vi "FGGA Serial Data Server & Recordingv4.0.vi"() -> ()   [LabVIEW 2014]
uses:
  <vilib>/Instr/_visa.llb/VISA Set IO Buffer Mask.ctl
  <vilib>/Instr/_visa.llb/VISA Flush IO Buffer Mask.ctl
  <vilib>/Platform/TimedLoop/XDataNode/timing_clust.ctl
  <vilib>/Platform/TimedLoop/XDataNode/nitl_modes.ctl
  <vilib>/Platform/TimedLoop/XDataNode/wakeup.ctl
  C:/Program Files (x86)/National Instruments/LabVIEW 2014/examples/Data Communication/Network Streams/Simple Network Streams/support/Network Stream Command.ctl
  <vilib>/Utility/error.llb/whitespace.ctl
  <vilib>/Instr/_visa.llb/VISA Configure Serial Port (Instr).vi
  <vilib>/Utility/tcp.llb/UDP Multicast Write-Only Open.vi
  <vilib>/platform/TimedLoop/XDataNode/XDataNode.xnode
  <vilib>/Platform/TimedLoop/XDataNode/XDNodeRunTimeDep.lvlib
panel:
  out "FGGA Pump":bool
  out "Flight Number":string
  out "Stop File Write":bool
  out "Default file name":string
  out "MFC":dbl[](array[numeric])
  out "FGGA restart":bool
  out "V4":bool
  out "V3":bool
  out "V2":bool
  out "V1":bool
  out "error out 2":errorcluster
  out "error out":errorcluster
  in  "MFC_1 SLPM set value":dbl
  out "Value Read":string
  out "status":bool
  in  "VISA resource name":refnum<visa-resource-name>="ASRL3::INSTR"
  in  "timeout (10sec) 2":u32=3000
  out "Labview_Viewer_UDP_Error_Out":errorcluster
  in  "Clear Display\nErrors":bool
  out "Data Processing":bool
  out "TCP Binary Packet":string
  out "UDP Time Stamp Offset":i32=1
  out "Data String":string
  out "UDP_ACSII_Out":string
  out "Serial error out":errorcluster
  out "SEPTIC TCP Error Out":errorcluster
  out "TCP packet\nSend To SEPTIC":bool
  out "FISH TCP Error Out":errorcluster
  out "TCP packet\nSend To FISH":bool
  out "UDP_Pack_num":u32
  out "UDP_Out Status":bool
  out "UDP_Out_Error Out":errorcluster
  out "Data Array":string[](array[string])
  out "RAW DATA":string
  in  "stop":bool
  in  "timeout (10sec)":u32=1500
  in  "VISA resource name":refnum<visa-resource-name>="ASRL7::INSTR"
  out "Number of times \nRead time out":u32
  out "Loop count":i32
  # "Date"
  # "Time"
  # "CH4"
  # "CO2"
  # "H2O"
  # "Cell Pressure"
  # "Cell Temperature"
  # "Spectral Flag"
  # "Ring Down Time (Laser A)"
  # "Ring Down Time (Laser B)"
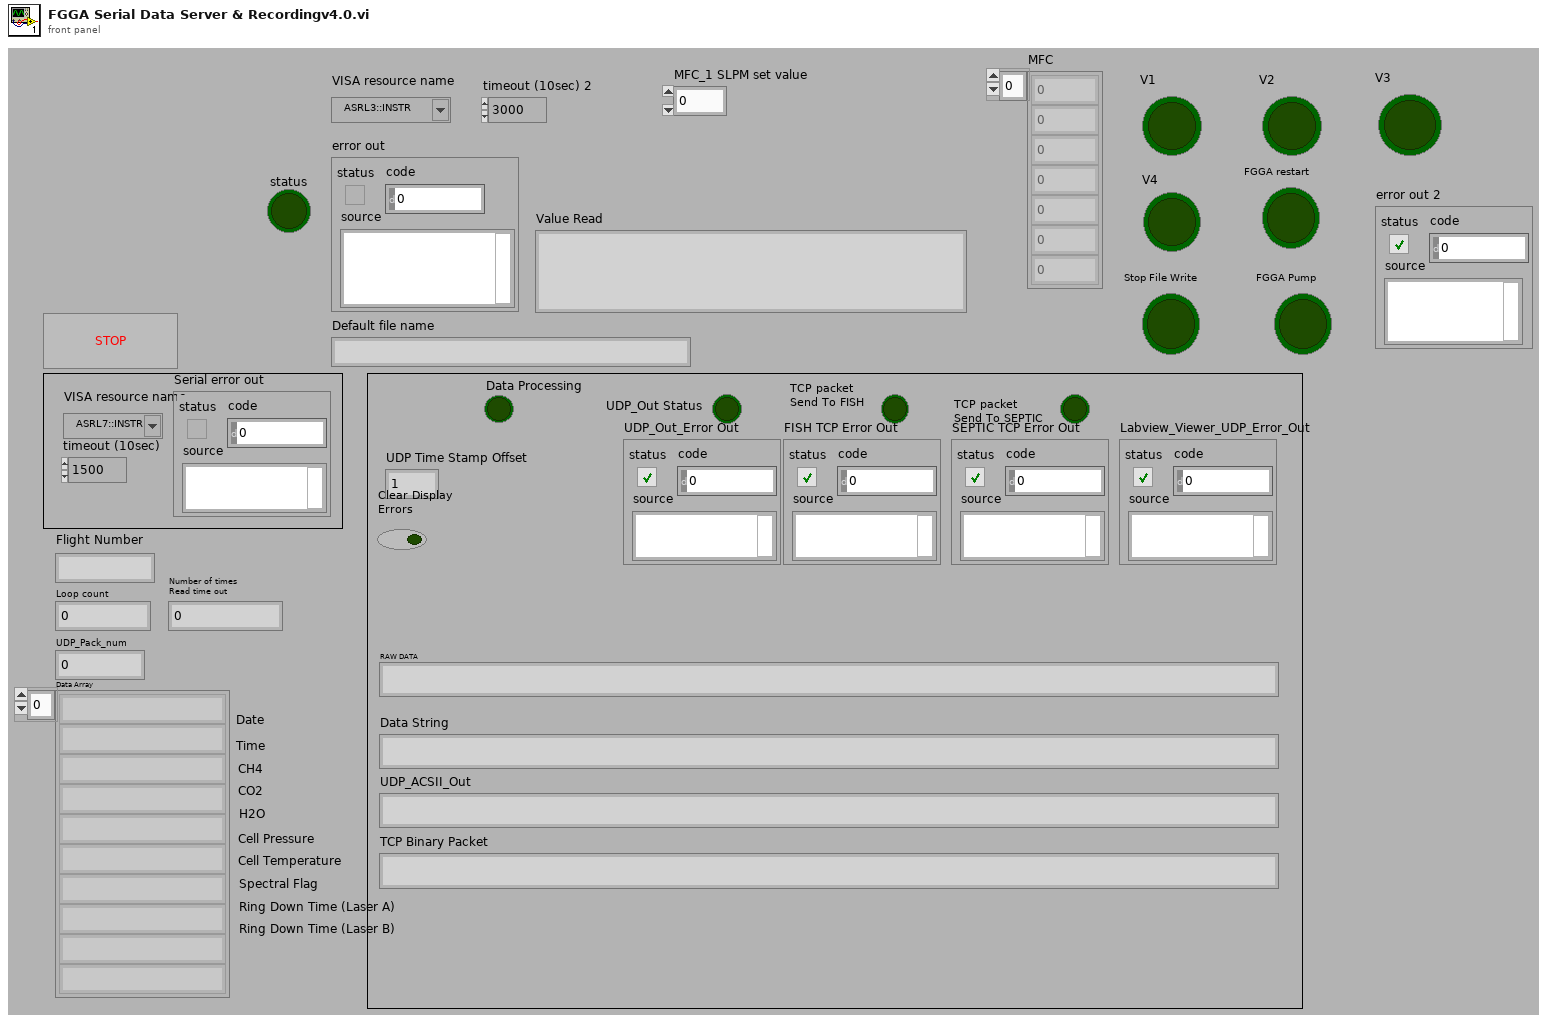
[diagram p1: front panel]
types:
  T1 = typedef "VISA Flush IO Buffer Mask.ctl" = u16
  T2 = typedef "VISA Set IO Buffer Mask.ctl" = u16
  T3 = typedef "XDNodeRunTimeDep.lvlib/timing_clust.ctl" = cluster{"Expected End [f-1]":u64, "Actual End [f-1]":u64, "Finished Late? [f-1]":bool, "Expected End [i-1]":u64, "Actual End [i-1]":u64, "Finished Late? [i-1]":bool, "Expected Start [i]":u64, "Actual Start [i]":u64, "Expected Start [f]":u64, "Actual Start [f]":u64, "Source Name":string, "Structure Name":string, "Period":i64, "Deadline":i64, "Offset":i64, "Start":i64, "Priority":i32, "Timeout":i32, "Mode":T4, "Wakeup Reason":T5, "Error":errorcluster, "Source Type":string, "Secondary Source Type":string, "Global End Time":u64, "Global Start Time":u64, "Frame Duration":u64, "Iteration Duration":u64, "Assigned CPU":i32, "I/O Scan Engine Mode":u32}
  T4 = typedef "XDNodeRunTimeDep.lvlib/nitl_modes.ctl" = enum32{"No Change", "Process missed periods, maintain original phase", "Discard missed periods, maintain original phase", "Process missed periods, ignore original phase", "Discard missed periods, ignore original phase"}
  T5 = typedef "XDNodeRunTimeDep.lvlib/wakeup.ctl" = enum32{"Normal", "Aborted", "Asynchronous wakeup", "Timing source error", "Timed loop error", "Timeout"}
  T6 = typedef "Network Stream Command.ctl" = cluster{"Message":string, "Message Data":variant}
  T7 = enum16{"open", "replace", "create", "open or create", "replace or create", "replace or create with confirmation"}
  T8 = typedef "whitespace.ctl" = u16
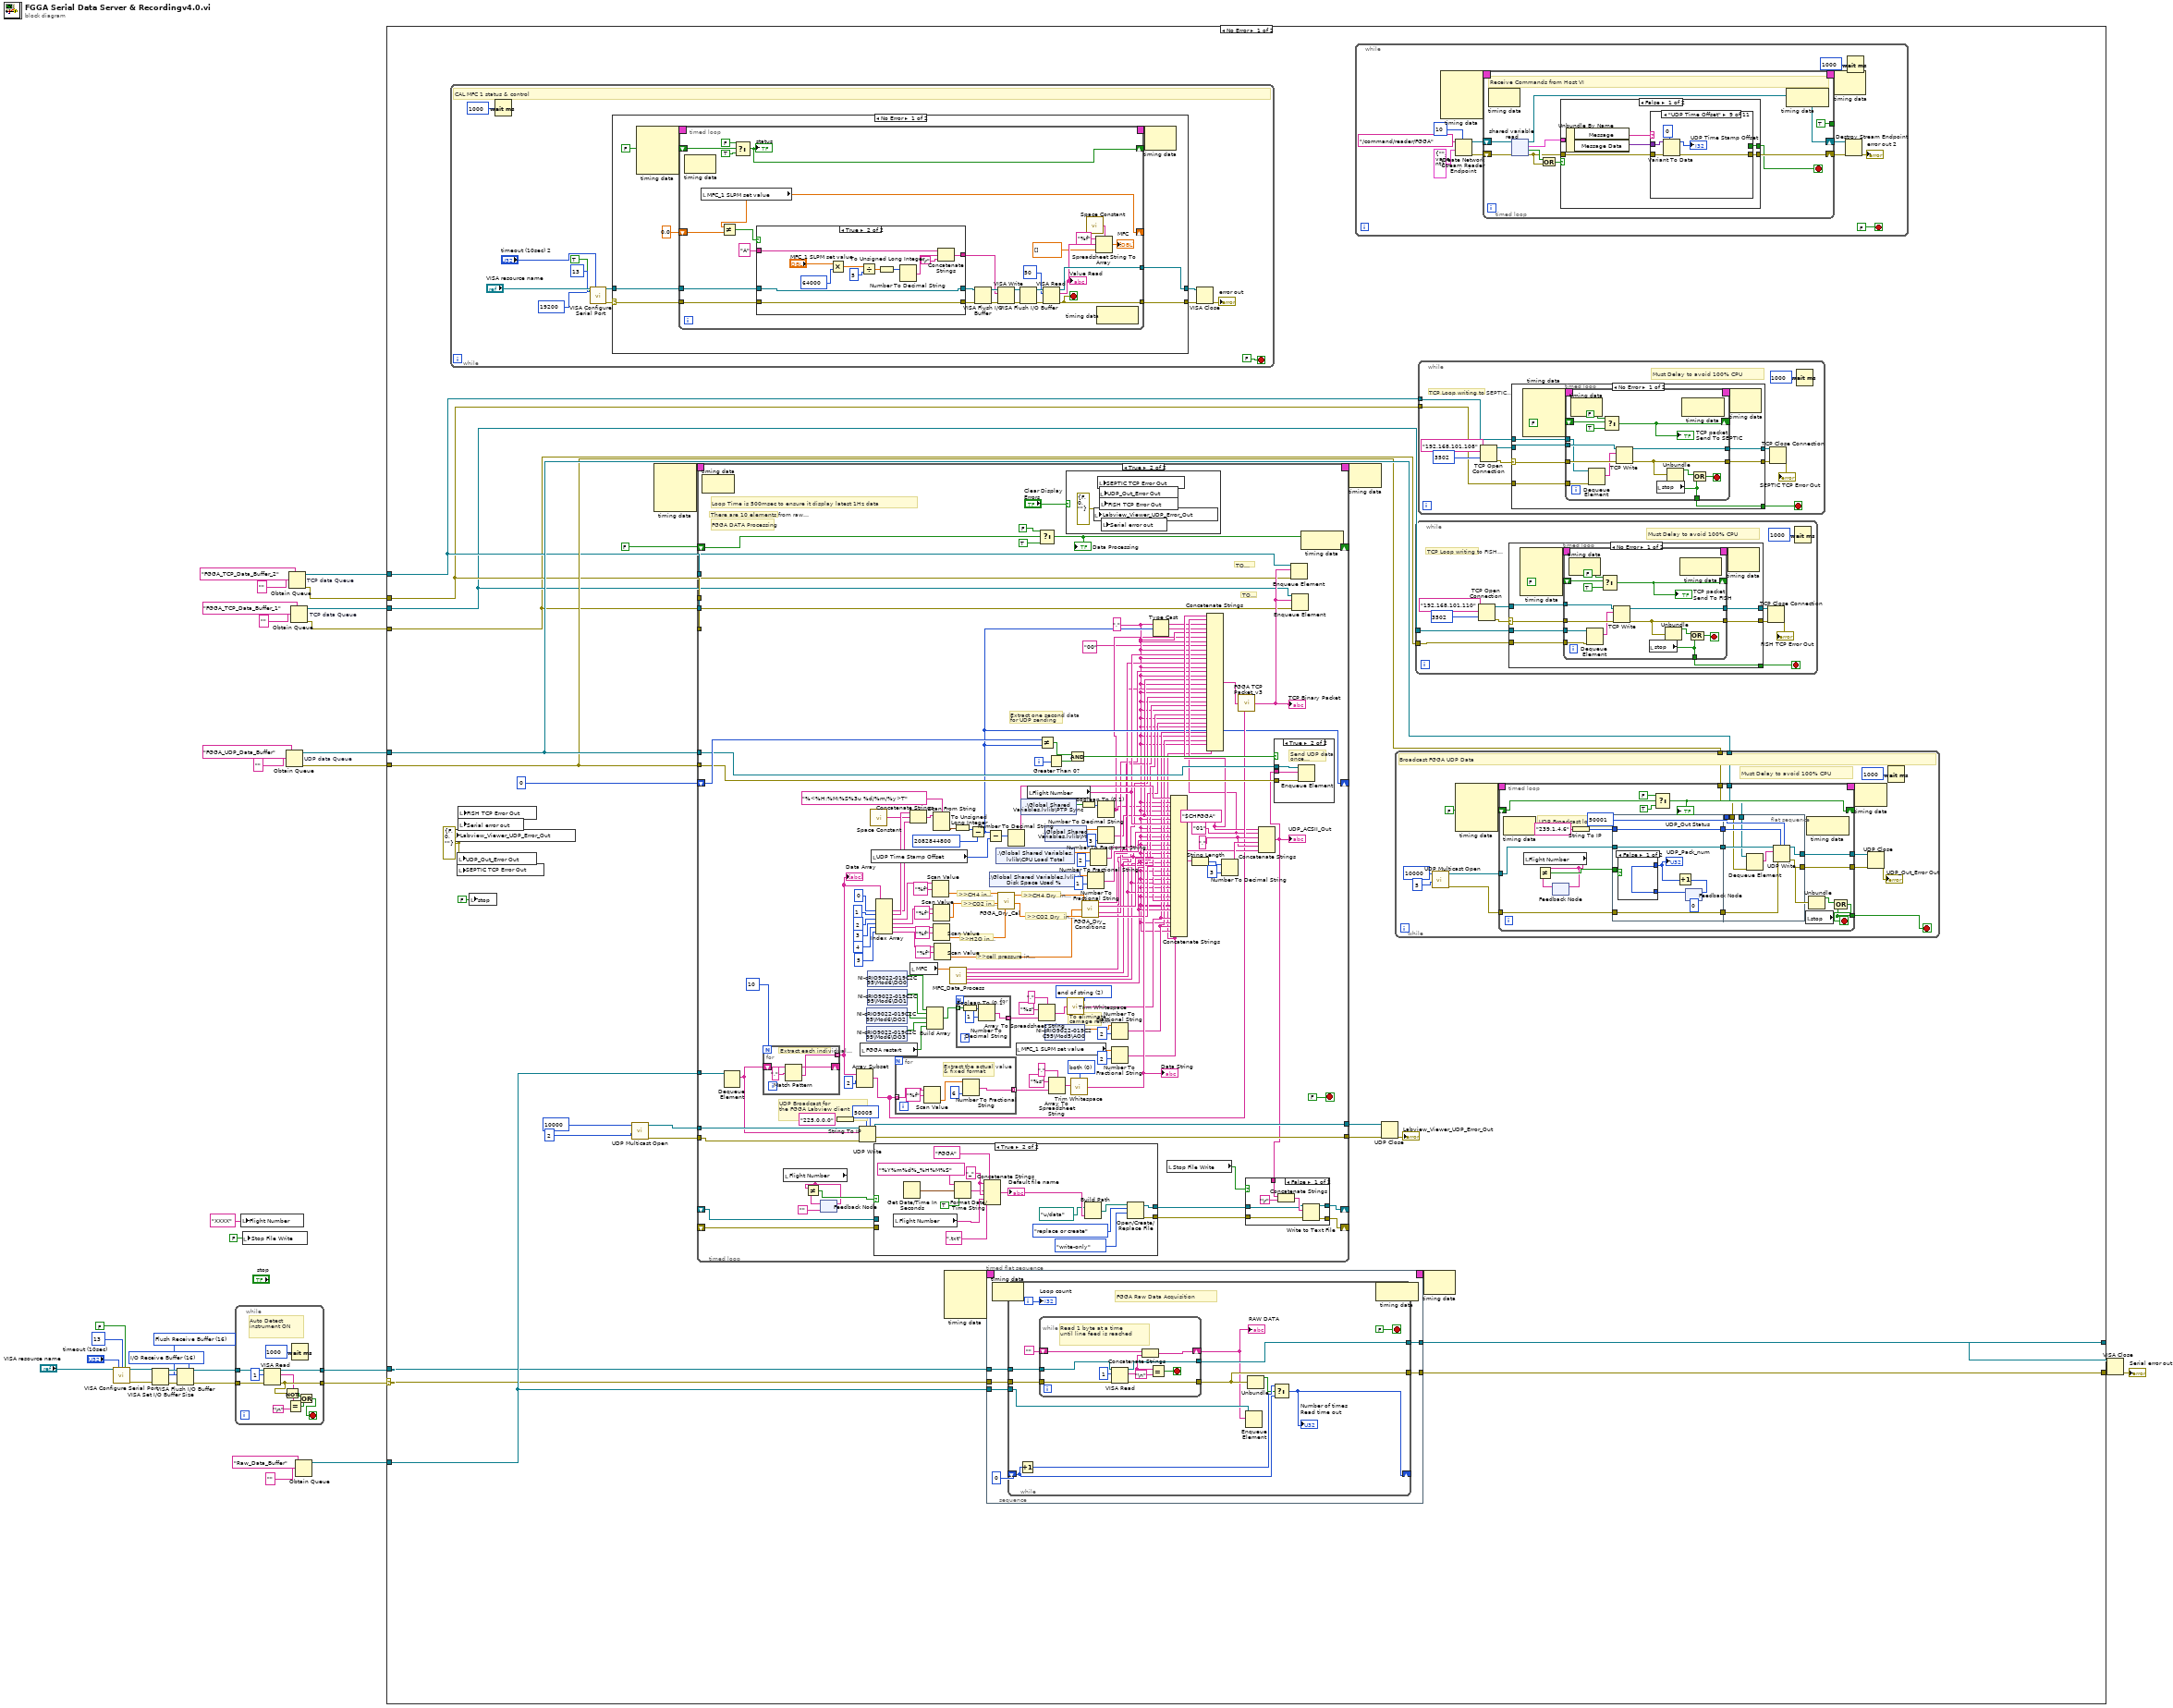
[diagram p0: block diagram]
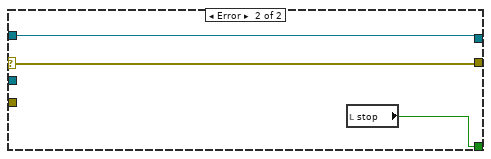
[diagram p2: hidden frame]
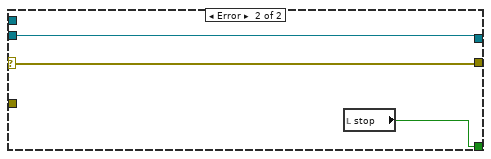
[diagram p3: hidden frame]
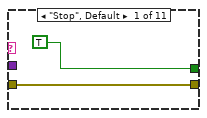
[diagram p4: hidden frame]
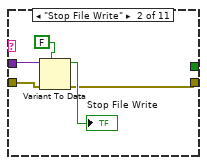
[diagram p5: hidden frame]
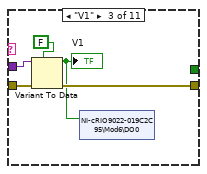
[diagram p6: hidden frame]
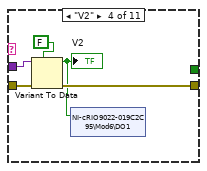
[diagram p7: hidden frame]
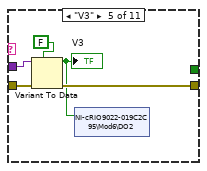
[diagram p8: hidden frame]
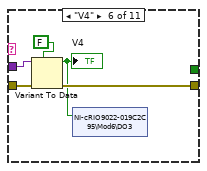
[diagram p9: hidden frame]
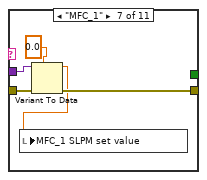
[diagram p10: hidden frame]
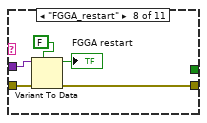
[diagram p11: hidden frame]
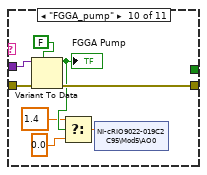
[diagram p12: hidden frame]
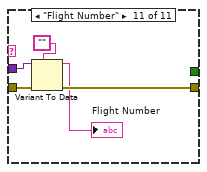
[diagram p13: hidden frame]
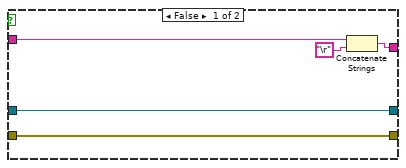
[diagram p15: hidden frame]
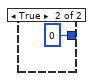
[diagram p17: hidden frame]
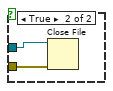
[diagram p19: hidden frame]
diagram:
  w9 = T1 16 items=["Flush Receive Buffer"=16, "Write Transmit Buffer to Device"=32, "Flush Receive Buffer (No I/O)"=64, "Flush Transmit Buffer"=128] ("Mask")
  w10 = T2 16 items=["I/O Receive Buffer"=16, "I/O Transmit Buffer"=32, "I/O Receive and Transmit Buffer"=48] ("Mask")
  n1 = call-poly "VISA Configure Serial Port"("VISA resource name"="VISA resource name", "timeout (10sec)"="timeout (10sec)", "termination char\n(0xA = '\\n' = LF)"=u8 13 ("termination char\n(0xA = '\\n' = LF)"), "Enable Termination\nChar (T)"=FALSE ("Enable Termination\nChar (T)")) -> ("VISA resource name out"=w8:refnum<visa-resource-name>, "error out"=w7:errorcluster)  [unwired: 10 in]
  n2 = VISA Set I/O Buffer Size(VISA resource name=w8, mask (16)=w10, error in (no error)=w7) -> (VISA resource name out=w11:refnum<visa-resource-name>, error out=w12:errorcluster)  [unwired: 1 in]
  n3 = VISA Flush I/O Buffer(VISA resource name=w11, mask (16)=w9, error in (no error)=w12) -> (VISA resource name out=w6:refnum<visa-resource-name>, error out=w5:errorcluster)
  n4 = while {
    tunnel: w6 -> [w45]
    tunnel: w5 -> [w44]
    tunnel: [w42] -> w4
    tunnel: [w41] -> w3
    stop <- w36 stop-if-true
    # "Auto Detect\ninstrument ON"
    n5 = VISA Read(VISA resource name=w45, byte count=u32 1, error in (no error)=w44) -> (VISA resource name out=w41:refnum<visa-resource-name>, read buffer=w39:string, error out=w42:errorcluster)  [unwired: 1 out]
    n6 = Not(x=w42) -> (.not. x?=w38:bool)
    n7 = Equal?(x=w39, y="\n") -> (x = y?=w37:bool)
    n8 = Wait (ms)(milliseconds to wait=u32 1000) -> ()  [unwired: 1 out]
    n9 = Or(x=w38, y=w37) -> (x .or. y?=w36:bool)
  }
  n10 = local write "Flight Number"("XXXX" ("Flight Number")) -> ()
  n11 = local write "Stop File Write"(FALSE ("Stop File Write")) -> ()
  n12 = Obtain Queue "UDP data Queue"(name (unnamed)="FGGA_UDP_Data_Buffer", element data type="") -> (queue out=w22:refnum<queue>, error out=w21:errorcluster)  [unwired: 3 in, 1 out]
  n13 = Obtain Queue "TCP data Queue"(name (unnamed)="FGGA_TCP_Data_Buffer_2", element data type="") -> (queue out=w16:refnum<queue>, error out=w15:errorcluster)  [unwired: 3 in, 1 out]
  n14 = Obtain Queue "TCP data Queue"(name (unnamed)="FGGA_TCP_Data_Buffer_1", element data type="") -> (queue out=w14:refnum<queue>, error out=w13:errorcluster)  [unwired: 3 in, 1 out]
  n15 = Obtain Queue(name (unnamed)="Raw_Data_Buffer", element data type="") -> (queue out=w28:refnum<queue>)  [unwired: 3 in, 2 out]
  n16 = case shown="No Error" w4 {
    selector: w4 -> [w48 w592]
    tunnel: w3 -> [w49 w593]
    tunnel: [w70 w593] -> w25
    tunnel: [w71 w592] -> w26
    tunnel: w28 -> [w67 _]
    tunnel: w22 -> [w65 _]
    tunnel: w21 -> [w64 _]
    tunnel: w16 -> [w63 _]
    tunnel: w15 -> [w62 _]
    tunnel: w14 -> [w61 _]
    tunnel: w13 -> [w60 _]
    frame No Error {
      w51 = errorcluster {"status"=FALSE, "code"=0, "source"=""} ("UDP Error Out")
      n17 = while {
        stop <- FALSE stop-if-true
        # "CAL MFC 1 status & control"
        n18 = Wait (ms)(milliseconds to wait=u32 1000) -> ()  [unwired: 1 out]
        n19 = call-poly "VISA Configure Serial Port"("VISA resource name"="VISA resource name", "timeout (10sec)"="timeout (10sec) 2", "termination char\n(0xA = '\\n' = LF)"=u8 13 ("termination char\n(0xA = '\\n' = LF)"), "Enable Termination\nChar (T)"=TRUE ("Enable Termination\nChar (T)"), "baud rate (9600)"=u32 19200) -> ("VISA resource name out"=w294:refnum<visa-resource-name>, "error out"=w290:errorcluster)  [unwired: 9 in]
        n20 = case shown="No Error" w290 {
          selector: w290 -> [w301 w351]
          tunnel: w294 -> [w302 w352]
          tunnel: [w300 w352] -> w293
          tunnel: [w299 w351] -> w292
          frame No Error {
            n21 = node-c288() -> (w297:T3)  [unwired: 4 in]
            n22 = timed-loop {
              tunnel: w302 -> [w325]
              tunnel: w301 -> [w323]
              tunnel: [w316] -> w300
              tunnel: [w311] -> w299
              shift-right: [w312] -> _
              shift-left: FALSE -> [w315]
              timing: w297 -> [_]
              timing-out: [_] -> w296
              shift-right: [w303] -> _
              shift-left: 0.0 -> [w305]
              stop <- w311 stop-if-true
              n23 = node-c288() -> ()  [unwired: 1 in, 1 out]
              n24 = local read "MFC_1 SLPM set value"() -> (w303:dbl)
              n25 = Not Equal?(x=w303, y=w305) -> (x != y?=w304:bool)
              n26 = Select(t=FALSE, s=w315, f=TRUE) -> (s? t:f=w312:bool)
              "status" <- w312
              n27 = case shown="True" w304 {
                tunnel: w325 -> [w333 w348]
                tunnel: [w333 w348] -> w324
                tunnel: w323 -> [w332 w347]
                tunnel: [w332 w347] -> w322
                tunnel: "A" -> [w336 w340]
                tunnel: [w334 w337] -> w320
                frame False {
                  n28 = Concatenate Strings(w336, "\r") -> (w334:string)
                }
                frame True {
                  n29 = Multiply(x="MFC_1 SLPM set value", y=u32 64000) -> (x*y=w344:dbl)
                  n30 = Divide(x=w344, y=u32 5) -> (x/y=w342:dbl)
                  n31 = To Unsigned Long Integer(number=w342) -> (unsigned 32bit integer=w341:u32)
                  n32 = Number To Decimal String(number=w341) -> (decimal integer string=w339:string)  [unwired: 1 in]
                  n33 = Concatenate Strings(w340, w339, "\r") -> (w337:string)
                }
              }
              n34 = VISA Flush I/O Buffer(VISA resource name=w324, error in (no error)=w322) -> (VISA resource name out=w327:refnum<visa-resource-name>, error out=w326:errorcluster)  [unwired: 1 in]
              n35 = VISA Write(VISA resource name=w327, write buffer=w320, error in (no error)=w326) -> (VISA resource name out=w319:refnum<visa-resource-name>, error out=w318:errorcluster)  [unwired: 1 out]
              n36 = VISA Flush I/O Buffer(VISA resource name=w319, error in (no error)=w318) -> (VISA resource name out=w329:refnum<visa-resource-name>, error out=w328:errorcluster)  [unwired: 1 in]
              n37 = VISA Read(VISA resource name=w329, byte count=u32 50, error in (no error)=w328) -> (VISA resource name out=w316:refnum<visa-resource-name>, read buffer=w310:string, error out=w311:errorcluster)  [unwired: 1 out]
              "Value Read" <- w310
              n38 = call <vilib>:"Space Constant.vi"() -> ("String"=w309:string)
              n39 = Spreadsheet String To Array(delimiter (Tab)=w309, format string="%f", spreadsheet string=w310, array type (2D Dbl)=dbl[] []) -> (array=→"MFC":dbl[])
              n40 = node-c288() -> ()  [unwired: 1 in, 1 out]
            }
            n41 = node-c288(w296) -> ()  [unwired: 1 out]
          }
          frame Error {
          }
        }
        n42 = VISA Close(VISA resource name=w293, error in (no error)=w292) -> (error out=→"error out":errorcluster)
      }
      n43 = local write "Labview_Viewer_UDP_Error_Out"(w51) -> ()
      n44 = local write "UDP_Out_Error Out"(w51) -> ()
      n45 = local write "SEPTIC TCP Error Out"(w51) -> ()
      n46 = local write "FISH TCP Error Out"(w51) -> ()
      n47 = local write "Serial error out"(w51) -> ()
      n48 = local write "stop"(FALSE ("stop")) -> ()
      n49 = call-poly <vilib>:"UDP Multicast Open.vi"("time-to-live (1)"=u16 2, "port"=u16 10000) -> ("error out"=w55:errorcluster, "connection ID"=w56:refnum<k16>)  [unwired: 8 in]
      n50 = node-c288() -> (w69:T3)  [unwired: 4 in]
      n51 = timed-loop {
        timing: w69 -> [_]
        timing-out: [_] -> w68
        tunnel: w67 -> [w544]
        tunnel: w65 -> [w500]
        tunnel: w64 -> [w499]
        shift-right: [w429] -> _
        shift-left: u32 0 -> [w503]
        tunnel: w63 -> [w496]
        tunnel: w62 -> [w495]
        tunnel: w61 -> [w494]
        tunnel: w60 -> [w493]
        shift-right: [w489] -> _
        shift-left: FALSE -> [w492]
        tunnel: w56 -> [w485]
        tunnel: w55 -> [w484]
        tunnel: [w483] -> w54
        tunnel: [w482] -> w53
        shift-right: [w469] -> _
        shift-left: _ -> [w461]
        shift-right: [w459] -> _
        shift-left: _ -> [w460]
        i -> [w502]
        stop <- FALSE stop-if-true
        w433 = T8 2 items=["both", "start of string", "end of string"] ("location (both)")
        w416 = ","
        w530 = T8 0 items=["both", "start of string", "end of string"] ("location (both)")
        w538 = ","
        w430 = "01"
        w431 = "$CHFGGA"
        # "To eliminate\ncarriage return"
        # ">>cell pressure in torr>>"
        # "UDP Broadcast for\nthe FGGA Labview client"
        # "There are 10 elements from raw packet"
        # "TO SEPTIC"
        # "TO FISH"
        # "Extract one second data\nfor UDP sending"
        # ">>CO2 Dry  in ppm>>"
        # ">>CH4 Dry  in ppb>>"
        # ">>H2O in ppm>>"
        # ">>CO2 in ppm>>"
        # ">>CH4 in ppm>>"
        # "Loop Time is 500msec to ensure it display latest 1Hz data"
        # "FGGA DATA Processing"
        n52 = node-c288() -> ()  [unwired: 1 in, 1 out]
        n53 = Dequeue Element(queue=w544) -> (element=w481:string)  [unwired: 2 in, 3 out]
        n54 = for {
          N: 10 -> [_]
          shift-right: [w586] -> _
          shift-left: w481 -> [w584]
          tunnel: [w585] -> w535 mode=indexing
          # "Extract each individual param"
          n55 = Match Pattern(string=w584, regular expression=",") -> (before substring=w585:string, after substring=w586:string)  [unwired: 1 in, 2 out]
        }
        "Data Array" <- w535
        n56 = local read "Flight Number"() -> (w458:string)
        n57 = feedback #1("" ("Flight Number")) -> (w466:string)
        n58 = Not Equal?(x=w458, y=w466) -> (x != y?=w464:bool)
        n59 = feedback-in #1(w458) -> ()
        n60 = String To IP(1:"225.0.0.0" ("name")) -> (0:w486:u32)
        n61 = Array Subset(array=w535, index=2) -> (w498:string[])  [unwired: 1 in]
        n62 = UDP Write(address=w486, port or service name=u16 50005, connection ID=w485, data in=w481, 8:w484) -> (error out=w482:errorcluster, 3:w483:refnum<k16>)  [unwired: 1 in]
        n63 = local read "FGGA restart"() -> (w443:bool)
        n64 = shared-variable "NI-cRIO9022-019C2C95\\Mod6\\DO2"() -> (w449:bool)  [unwired: 1 in, 1 out]
        n65 = shared-variable "NI-cRIO9022-019C2C95\\Mod6\\DO3"() -> (w448:bool)  [unwired: 1 in, 1 out]
        n66 = shared-variable "NI-cRIO9022-019C2C95\\Mod6\\DO0"() -> (w451:bool)  [unwired: 1 in, 1 out]
        n67 = shared-variable "NI-cRIO9022-019C2C95\\Mod6\\DO1"() -> (w450:bool)  [unwired: 1 in, 1 out]
        n68 = call <vilib>:"Space Constant.vi"() -> ("String"=w513:string)
        n69 = local read "UDP Time Stamp Offset"() -> (w432:i32)
        n70 = case shown="True" w464 {
          tunnel: [w550 w552] -> w463
          tunnel: [w549 w551] -> w462
          tunnel: w461 -> [w550 _]
          tunnel: w460 -> [w549 _]
          frame False {
          }
          frame True {
            w558 = "_" ("string")
            n71 = local read "Flight Number"() -> (w565:string)
            n72 = Get Date/Time In Seconds() -> (seconds since 1Jan1904=w553:timestamp)
            n73 = Format Date/Time String(time format string (%c)="%Y%m%d%_%H%M%S", seconds (now)=w553, UTC format=TRUE) -> (date/time string=w555:string)
            n74 = Concatenate Strings("FGGA" ("string"), w558, w555, w558, w565, ".txt" ("string")) -> (w560:string)
            "Default file name" <- w560
            n75 = Build Path(base path=path "u:/data", name or relative path=w560) -> (appended path=w564:path)
            n76 = Open/Create/Replace File(file path (use dialog)=w564, operation (0:open)=T7."replace or create", access (0:read/write)=enum16{"read/write", "read-only", "write-only"}."write-only") -> (refnum out=w552:refnum<file>, error out=w551:errorcluster)  [unwired: 3 in, 1 out]
          }
        }
        n77 = Index Array(array=w535, index #1=0 ("index"), index #2=1 ("index"), index #3=2 ("index"), index #4=3 ("index"), index #5=4 ("index"), index #6=5 ("index")) -> (element #1=w512:string, element #2=w514:string, element #3=w518:string, element #4=w517:string, element #5=w516:string, element #6=w474:string)
        n78 = for {
          tunnel: w498 -> [w582] mode=indexing
          tunnel: [w579] -> w528 mode=indexing
          # "Extract the actual value\n& fixed format"
          n79 = Scan Value(string=w582, format string="%f") -> (value=w580:dbl)  [unwired: 1 in, 1 out]
          n80 = Number To Fractional String(number=w580, precision (6)=i16 6) -> (F-format string=w579:string)  [unwired: 2 in]
        }
        n81 = Concatenate Strings(w514, w513, w512) -> (w511:string)
        n82 = local read "MFC"() -> (w470:dbl[])
        n83 = Build Array(w451, w450, w449, w448, w443) -> (w447:bool[])
        n84 = Scan Value(string=w518, format string="%f") -> (value=w520:dbl)  [unwired: 1 in, 1 out]
        n85 = Scan Value(string=w517, format string="%f") -> (value=w519:dbl)  [unwired: 1 in, 1 out]
        n86 = Scan From String(format string="%<%H:%M:%S%3u %d/%m/%y>T", input string=w511) -> (output 1=w508:timestamp)  [unwired: 3 in, 3 out]
        n87 = Scan Value(string=w516, format string="%f") -> (value=w471:dbl)  [unwired: 1 in, 1 out]
        n88 = Scan Value(string=w474, format string="%f") -> (value=w472:dbl)  [unwired: 1 in, 1 out]
        n89 = call "MFC_Data_Process.vi"("MFC"=w470) -> ("MFC Absolute Pressure"=w423:string, "MFC Temperature"=w422:string, "MFC Volumetric Flow"=w421:string, "MFC Mass Flow"=w420:string, "MFC Set Point"=w419:string)  [unwired: 10 in]
        n90 = To Unsigned Long Integer(number=w508) -> (unsigned 32bit integer=w509:u32)
        n91 = for {
          tunnel: w447 -> [w547] mode=indexing
          tunnel: [w546] -> w444 mode=indexing
          n92 = Boolean To (0,1)(Boolean=w547) -> (0, 1=w548:i16)
          n93 = Number To Decimal String(number=w548, width (-)=i16 1) -> (decimal integer string=w546:string)
        }
        n94 = Subtract(x=w509, y=u32 2082844800) -> (x-y=w429:u32)
        n95 = Subtract(x=w429, y=w432) -> (x-y=w506:u32)
        n96 = shared-variable ".\\Global Shared Variables.lvlib\\Disk Space Used %"() -> (w436:dbl)  [unwired: 1 in, 1 out]
        n97 = shared-variable ".\\Global Shared Variables.lvlib\\CPU Load Total"() -> (w457:dbl)  [unwired: 1 in, 1 out]
        n98 = call "FGGA_Dry_Cal.vi"("H2O"=w471, "CO2_Wet"=w519, "CH4_Wet"=w520) -> ("CO2_Dry"=w476:dbl, "CH4_Dry"=w478:dbl)  [unwired: 7 in]
        n99 = Number To Decimal String(number=w506) -> (decimal integer string=w507:string)  [unwired: 1 in]
        n100 = local read "MFC_1 SLPM set value"() -> (w439:dbl)
        n101 = shared-variable ".\\Global Shared Variables.lvlib\\PTP Sync"() -> (w452:bool)  [unwired: 1 in, 1 out]
        n102 = local read "Flight Number"() -> (w427:string)
        n103 = Array To Spreadsheet String(delimiter (Tab)=",", array=w444, 3:"%s" ("format string")) -> (spreadsheet string=w434:string)
        n104 = Select(t=FALSE, s=w492, f=TRUE) -> (s? t:f=w489:bool)
        "Data Processing" <- w489
        n105 = Not Equal?(x=w503, y=w429) -> (x != y?=w504:bool)
        n106 = shared-variable ".\\Global Shared Variables.lvlib\\MFM"() -> (w455:dbl)  [unwired: 1 in, 1 out]
        n107 = shared-variable "NI-cRIO9022-019C2C95\\Mod5\\AO0"() -> (w441:dbl)  [unwired: 1 in, 1 out]
        n108 = Greater Than 0?(x=w502) -> (x > 0?=w505:bool)
        n109 = Array To Spreadsheet String(delimiter (Tab)=",", array=w528, 3:"%s" ("format string")) -> (spreadsheet string=w529:string)
        n110 = case shown="True" "Clear Display\nErrors" {
          frame False {
          }
          frame True {
            w575 = errorcluster {"status"=FALSE, "code"=0, "source"=""} ("UDP Error Out")
            n111 = local write "Labview_Viewer_UDP_Error_Out"(w575) -> ()
            n112 = local write "SEPTIC TCP Error Out"(w575) -> ()
            n113 = local write "UDP_Out_Error Out"(w575) -> ()
            n114 = local write "FISH TCP Error Out"(w575) -> ()
            n115 = local write "Serial error out"(w575) -> ()
          }
        }
        n116 = call <vilib>:"Trim Whitespace.vi"("string"=w434, "location (both)"=w433) -> ("trimmed string"=w418:string)
        n117 = call <vilib>:"Trim Whitespace.vi"("string"=w529, "location (both)"=w530) -> ("trimmed string"=w527:string)
        "Data String" <- w527
        n118 = Compound Arithmetic op=AND(w504, w505) -> (w501:bool)
        n119 = Boolean To (0,1)(Boolean=w452) -> (0, 1=w453:i16)
        n120 = call "FGGA_Dry_Conditions.vi"("CH4_Dry"=w478, "Pressure"=w472, "CO2_Dry"=w476) -> ("CH4_Dry_TCP"=w426:string, "CH4_Dry_UDP"=w480:string, "CO2_Dry_TCP"=w425:string, "CO2_Dry_UDP"=w479:string)  [unwired: 9 in]
        n121 = Number To Fractional String(number=w436, precision (6)=i16 1) -> (F-format string=w435:string)  [unwired: 2 in]
        n122 = Number To Fractional String(number=w457, precision (6)=i16 2) -> (F-format string=w438:string)  [unwired: 2 in]
        n123 = Number To Decimal String(number=w453) -> (decimal integer string=w413:string)  [unwired: 1 in]
        n124 = Number To Fractional String(number=w455, precision (6)=i16 3) -> (F-format string=w424:string)  [unwired: 2 in]
        n125 = Number To Fractional String(number=w441, precision (6)=i16 2) -> (F-format string=w417:string)  [unwired: 2 in]
        n126 = Number To Fractional String(number=w439, precision (6)=i16 2) -> (F-format string=w415:string)  [unwired: 2 in]
        n127 = Type Cast(x=w429) -> (*(type *) &x=w428:string)  [unwired: 1 in]
        n128 = local read "Stop File Write"() -> (w467:bool)
        n129 = Concatenate Strings(w507, w416, w413, w416, w424, w416, w427, w416, w438, w416, w435, w416, w527, w416, w480, w416, w479, w416, w423, w416, w422, w416, w421, w416, w420, w416, w419, w416, w418, w416, w417, w416, w415) -> (w537:string)
        n130 = String Length(string=w537) -> (length=w541:i32)
        n131 = Concatenate Strings(w431, w430, w416, w428, w416, w413, w416, "00", w416, w427, w416, w426, w416, w425, w416, w424, w416, w423, w416, w422, w416, w421, w416, w420, w416, w419, w416, w418, w416, w417, w416, w415) -> (w414:string)
        n132 = Number To Decimal String(number=w541, width (-)=i16 3) -> (decimal integer string=w539:string)
        n133 = call "FGGA TCP Packet_v3.vi"("TCP Packet In"=w414, "Data Array"=w498) -> ("TCP Binary Packet"=w497:string)  [unwired: 13 in]
        "TCP Binary Packet" <- w497
        n134 = Concatenate Strings(w431, w430, w538, w539, w538, w537) -> (w468:string)
        "UDP_ACSII_Out" <- w468
        n135 = case shown="False" w467 {
          tunnel: w468 -> [w572 _]
          tunnel: [w569 _] -> w469
          tunnel: w463 -> [w568 w574]
          tunnel: w462 -> [w567 w573]
          tunnel: [w566 _] -> w459
          frame False {
            n136 = Concatenate Strings(w572, "\r") -> (w570:string)
            n137 = Write to Text File(file (use dialog)=w568, text=w570, error in=w567) -> (refnum out=w569:refnum<file>, error out=w566:errorcluster)  [unwired: 2 out]
          }
          frame True {
            n138 = Close File(refnum=w574, error in=w573) -> ()  [unwired: 2 out]
          }
        }
        n139 = case shown="True" w501 {
          tunnel: w468 -> [_ w578]
          tunnel: w500 -> [_ w577]
          tunnel: w499 -> [_ w576]
          frame False {
          }
          frame True {
            # "Send UDP data once\na second"
            n140 = Enqueue Element(queue=w577, element=w578, error in (no error)=w576) -> ()  [unwired: 1 in, 3 out]
          }
        }
        n141 = Enqueue Element(queue=w496, element=w497, error in (no error)=w495) -> ()  [unwired: 1 in, 3 out]
        n142 = Enqueue Element(queue=w494, element=w497, error in (no error)=w493) -> ()  [unwired: 1 in, 3 out]
        n143 = node-c288() -> ()  [unwired: 1 in, 1 out]
      }
      n144 = node-c288() -> (w47:T3)  [unwired: 4 in]
      n145 = timed-sequence {
        timing: w47 -> [_]
        timing-out: [_] -> w46
        tunnel: [w160] -> w71
        tunnel: [w159] -> w70
        tunnel: w67 -> [w158]
        tunnel: w49 -> [w157]
        tunnel: w48 -> [w156]
        n146 = timed-flat-sequence {
          tunnel: [w166] -> w160
          tunnel: [w165] -> w159
          tunnel: w158 -> [w163]
          tunnel: w157 -> [w162]
          tunnel: w156 -> [w161]
          n147 = node-c288() -> ()  [unwired: 1 in, 1 out]
          n148 = while {
            tunnel: w162 -> [w179]
            tunnel: w161 -> [w178]
            tunnel: [w177] -> w166
            shift-right: [w173] -> _
            shift-left: u32 0 -> [w174]
            tunnel: [w176] -> w165
            tunnel: w163 -> [w170]
            i -> [w175]
            stop <- FALSE stop-if-true
            # "FGGA Raw Data Acquisition"
            n149 = Increment(x=w174) -> (x+1=w172:u32)
            n150 = while {
              tunnel: [w189] -> w176
              tunnel: [w188] -> w177
              tunnel: w179 -> [w187]
              tunnel: w178 -> [w186]
              shift-right: [w184] -> w169
              shift-left: "" -> [w185]
              stop <- w181 stop-if-true
              # "Read 1 byte at a time \nuntil line feed is reached"
              n151 = VISA Read(VISA resource name=w187, byte count=u32 1, error in (no error)=w186) -> (VISA resource name out=w189:refnum<visa-resource-name>, read buffer=w183:string, error out=w188:errorcluster)  [unwired: 1 out]
              n152 = Concatenate Strings(w185, w183) -> (w184:string)
              n153 = Equal?(x=w183, y="\n") -> (x = y?=w181:bool)
            }
            "RAW DATA" <- w169
            n154 = Enqueue Element(queue=w170, element=w169) -> ()  [unwired: 2 in, 3 out]
            n155 = Unbundle(w177) -> ("status"=w168:bool)  [unwired: 2 out]
            n156 = Select(t=w172, s=w168, f=w174) -> (s? t:f=w173:u32)
            "Number of times \nRead time out" <- w173
            "Loop count" <- w175
          }
          n157 = node-c288() -> ()  [unwired: 1 in, 1 out]
        }
      }
      n158 = node-c288(w68) -> ()  [unwired: 1 out]
      n159 = while {
        stop <- FALSE stop-if-true
        n160 = node-c288() -> (w195:T3)  [unwired: 4 in]
        n161 = Create Network Stream Reader Endpoint(7:10 ("reader buffer size"), 9:T6 {"Message"="", "Message Data"=variant} ("Message Cluster"), 11:"/command/reader/FGGA" ("reader url")) -> (0:w201:errorcluster, 3:w202:refnum<k21>)  [unwired: 4 in]
        n162 = timed-loop "Host->Target Command Reader" {
          shift-right: [w212] -> w199
          shift-left: w201 -> [w215]
          shift-right: [w213] -> w198
          shift-left: w202 -> [w214]
          tunnel: [TRUE] -> _
          timing: w195 -> [_]
          timing-out: [_] -> w194
          stop <- w206 stop-if-true
          # "Receive Commands from Host VI"
          n163 = node-c288() -> ()  [unwired: 1 in, 1 out]
          n164 = shared-variable-read(w214, w215) -> (w213:refnum<k21>, w208:errorcluster, w210:bool, w211:T6)  [unwired: 1 in]
          n165 = Or(x=w210, y=w208) -> (x .or. y?=w209:bool)
          n166 = case shown="False" w209 {
            selector: w209 -> [_ w279]
            tunnel: w208 -> [w223 w280]
            tunnel: [w222 w280] -> w212
            tunnel: w211 -> [w220 _]
            tunnel: [w221 w279] -> w206
            frame False {
              n167 = Unbundle By Name(w220) -> ("Message"=w219:string, "Message Data"=w218:variant)
              n168 = case shown="\"UDP Time Offset\"" w219 {
                tunnel: w223 -> [w225 w230 w235 w240 w245 w250 w255 w260 w265 w273 w278]
                tunnel: [w225 w226 w234 w239 w244 w249 w254 w259 w264 w272 w277] -> w222
                tunnel: w218 -> [_ w229 w233 w238 w243 w248 w253 w258 w263 w271 w276]
                tunnel: [TRUE _ _ _ _ _ _ _ _ _ _] -> w221
                frame "Stop", Default {
                }
                frame "Stop File Write" {
                  n169 = Variant To Data(error in=w230, type=FALSE, Variant=w229) -> (data=→"Stop File Write":bool, error out=w226:errorcluster)
                }
                frame "V1" {
                  n170 = Variant To Data(error in=w235, type=FALSE, Variant=w233) -> (data=w231:bool, error out=w234:errorcluster)
                  "V1" <- w231
                  n171 = shared-variable "NI-cRIO9022-019C2C95\\Mod6\\DO0"(w231) -> ()  [unwired: 1 in, 1 out]
                }
                frame "V2" {
                  n172 = Variant To Data(error in=w240, type=FALSE, Variant=w238) -> (data=w236:bool, error out=w239:errorcluster)
                  "V2" <- w236
                  n173 = shared-variable "NI-cRIO9022-019C2C95\\Mod6\\DO1"(w236) -> ()  [unwired: 1 in, 1 out]
                }
                frame "V3" {
                  n174 = Variant To Data(error in=w245, type=FALSE, Variant=w243) -> (data=w241:bool, error out=w244:errorcluster)
                  "V3" <- w241
                  n175 = shared-variable "NI-cRIO9022-019C2C95\\Mod6\\DO2"(w241) -> ()  [unwired: 1 in, 1 out]
                }
                frame "V4" {
                  n176 = Variant To Data(error in=w250, type=FALSE, Variant=w248) -> (data=w246:bool, error out=w249:errorcluster)
                  "V4" <- w246
                  n177 = shared-variable "NI-cRIO9022-019C2C95\\Mod6\\DO3"(w246) -> ()  [unwired: 1 in, 1 out]
                }
                frame "MFC_1" {
                  n178 = Variant To Data(error in=w255, type=0.0, Variant=w253) -> (data=w251:dbl, error out=w254:errorcluster)
                  n179 = local write "MFC_1 SLPM set value"(w251) -> ()
                }
                frame "FGGA_restart" {
                  n180 = Variant To Data(error in=w260, type=FALSE, Variant=w258) -> (data=→"FGGA restart":bool, error out=w259:errorcluster)
                }
                frame "UDP Time Offset" {
                  n181 = Variant To Data(error in=w265, type=0, Variant=w263) -> (data=→"UDP Time Stamp Offset":i32, error out=w264:errorcluster)
                }
                frame "FGGA_pump" {
                  n182 = Variant To Data(error in=w273, type=FALSE, Variant=w271) -> (data=w268:bool, error out=w272:errorcluster)
                  "FGGA Pump" <- w268
                  n183 = Select(t=1.4 ("f"), s=w268, f=0.0 ("t")) -> (s? t:f=w269:dbl)
                  n184 = shared-variable "NI-cRIO9022-019C2C95\\Mod5\\AO0"(w269) -> ()  [unwired: 1 in, 1 out]
                }
                frame "Flight Number" {
                  n185 = Variant To Data(error in=w278, type="", Variant=w276) -> (data=→"Flight Number":string, error out=w277:errorcluster)
                }
              }
            }
            frame True {
            }
          }
          n186 = node-c288() -> ()  [unwired: 1 in, 1 out]
        }
        n187 = node-c288(w194) -> ()  [unwired: 1 out]
        n188 = Destroy Stream Endpoint(8:w199, 11:w198) -> (0:→"error out 2":errorcluster)
        n189 = Wait (ms)(milliseconds to wait=u32 1000) -> ()  [unwired: 1 out]
      }
      n190 = UDP Close(connection ID=w54, 8:w53) -> (error out=→"Labview_Viewer_UDP_Error_Out":errorcluster)  [unwired: 1 out]
      n191 = while {
        tunnel: w65 -> [w355]
        tunnel: w64 -> [w354]
        stop <- w356 stop-if-true
        # "Must Delay to avoid 100% CPU"
        # "Broadcast FGGA UDP Data"
        n192 = call-poly <vilib>:"UDP Multicast Open.vi"("time-to-live (1)"=u16 5, "port"=u16 10000) -> ("error out"=w363:errorcluster, "connection ID"=w364:refnum<k16>)  [unwired: 8 in]
        n193 = node-c288() -> (w366:T3)  [unwired: 4 in]
        n194 = timed-loop {
          tunnel: w364 -> [w387]
          tunnel: w363 -> [w386]
          timing: w366 -> [_]
          timing-out: [_] -> w365
          shift-right: [w375] -> _
          shift-left: FALSE -> [w378]
          tunnel: [w374] -> w358
          tunnel: [w372] -> w357
          tunnel: [w370] -> w356
          tunnel: w355 -> [w368]
          tunnel: w354 -> [w367]
          stop <- w371 stop-if-true
          # "UDP Broadcast loop"
          n195 = node-c288() -> ()  [unwired: 1 in, 1 out]
          n196 = local read "Flight Number"() -> (w369:string)
          n197 = feedback-in #2(w369) -> ()
          n198 = feedback #2() -> (w380:string)  [unwired: 1 in]
          n199 = Not Equal?(x=w369, y=w380) -> (x != y?=w379:bool)
          n200 = String To IP(1:"239.1.4.6" ("name")) -> (0:w384:u32)
          n201 = flat-sequence {
            tunnel: w384 -> [w394]
            tunnel: w386 -> [w395]
            tunnel: w387 -> [w396]
            tunnel: [w396] -> w383
            tunnel: [w395] -> w382
            tunnel: [w394] -> w381
            tunnel: w379 -> [w393]
            tunnel: u16 50001 ("port or service name") -> [w407]
            tunnel: w383 -> [w406]
            tunnel: w382 -> [w405]
            tunnel: w381 -> [w404]
            tunnel: [w403] -> w374
            tunnel: [w402] -> w372
            tunnel: w368 -> [w400]
            tunnel: w367 -> [w399]
            frame #0 {
              n202 = feedback #3(u32 0) -> (w390:u32)
              n203 = case shown="False" w393 {
                tunnel: w390 -> [w397 _]
                tunnel: [w397 u32 0] -> w389
                frame False {
                }
                frame True {
                }
              }
              "UDP_Pack_num" <- w389
              n204 = Increment(x=w389) -> (x+1=w391:u32)
              n205 = feedback-in #3(w391) -> ()
            }
            frame #1 {
              n206 = Dequeue Element(queue=w400, error in (no error)=w399) -> (element=w401:string)  [unwired: 1 in, 3 out]
              n207 = UDP Write(address=w404, port or service name=w407, connection ID=w406, data in=w401, 8:w405) -> (error out=w402:errorcluster, 3:w403:refnum<k16>)  [unwired: 1 in]
            }
          }
          n208 = Select(t=FALSE, s=w378, f=TRUE) -> (s? t:f=w375:bool)
          "UDP_Out Status" <- w375
          n209 = local read "stop"() -> (w370:bool)
          n210 = node-c288() -> ()  [unwired: 1 in, 1 out]
          n211 = Unbundle(w372) -> ("status"=w373:bool)  [unwired: 2 out]
          n212 = Compound Arithmetic op=OR(w373, w370) -> (w371:bool)
        }
        n213 = node-c288(w365) -> ()  [unwired: 1 out]
        n214 = UDP Close(connection ID=w358, 8:w357) -> (error out=→"UDP_Out_Error Out":errorcluster)  [unwired: 1 out]
        n215 = Wait (ms)(milliseconds to wait=u32 1000) -> ()  [unwired: 1 out]
      }
      n216 = while {
        tunnel: w61 -> [w74]
        tunnel: w60 -> [w73]
        stop <- w77 stop-if-true
        # "Must Delay to avoid 100% CPU"
        # "TCP Loop writing to FISH Tank"
        n217 = TCP Open Connection(address="192.168.101.110", remote port or service name=u16 3502) -> (connection ID=w80:refnum<k5>, error out=w75:errorcluster)  [unwired: 3 in]
        n218 = case shown="No Error" w75 {
          selector: w75 -> [w85 w112]
          tunnel: w80 -> [w90 w113]
          tunnel: [w89 w113] -> w79
          tunnel: [w88 w112] -> w78
          tunnel: [w87 w111] -> w77
          tunnel: w74 -> [w84 _]
          tunnel: w73 -> [w83 _]
          frame No Error {
            n219 = node-c288() -> (w92:T3)  [unwired: 4 in]
            n220 = timed-loop {
              tunnel: w90 -> [w106]
              tunnel: w85 -> [w105]
              tunnel: [w104] -> w89
              tunnel: [w103] -> w88
              tunnel: [w95] -> w87
              shift-right: [w97] -> _
              shift-left: FALSE -> [w100]
              timing: w92 -> [_]
              timing-out: [_] -> w91
              tunnel: w84 -> [w94]
              tunnel: w83 -> [w93]
              stop <- w101 stop-if-true
              n221 = node-c288() -> ()  [unwired: 1 in, 1 out]
              n222 = Dequeue Element(queue=w94, error in (no error)=w93) -> (element=w96:string)  [unwired: 1 in, 3 out]
              n223 = Select(t=FALSE, s=w100, f=TRUE) -> (s? t:f=w97:bool)
              "TCP packet\nSend To FISH" <- w97
              n224 = TCP Write(connection ID=w106, data in=w96, error in (no error)=w105) -> (connection ID out=w104:refnum<k5>, error out=w103:errorcluster)  [unwired: 1 in, 1 out]
              n225 = local read "stop"() -> (w95:bool)
              n226 = Unbundle(w103) -> ("status"=w102:bool)  [unwired: 2 out]
              n227 = node-c288() -> ()  [unwired: 1 in, 1 out]
              n228 = Compound Arithmetic op=OR(w102, w95) -> (w101:bool)
            }
            n229 = node-c288(w91) -> ()  [unwired: 1 out]
          }
          frame Error {
            n230 = local read "stop"() -> (w111:bool)
          }
        }
        n231 = TCP Close Connection(connection ID=w79, error in (no error)=w78) -> (error out=→"FISH TCP Error Out":errorcluster)  [unwired: 1 in, 1 out]
        n232 = Wait (ms)(milliseconds to wait=u32 1000) -> ()  [unwired: 1 out]
      }
      n233 = while {
        tunnel: w63 -> [w116]
        tunnel: w62 -> [w115]
        stop <- w119 stop-if-true
        # "Must Delay to avoid 100% CPU"
        # "TCP Loop writing to SEPTIC Tank"
        n234 = TCP Open Connection(address="192.168.101.108", remote port or service name=u16 3502) -> (connection ID=w122:refnum<k5>, error out=w117:errorcluster)  [unwired: 3 in]
        n235 = case shown="No Error" w117 {
          selector: w117 -> [w127 w154]
          tunnel: w122 -> [w132 w155]
          tunnel: [w131 w155] -> w121
          tunnel: [w130 w154] -> w120
          tunnel: [w129 w153] -> w119
          tunnel: w116 -> [w126 _]
          tunnel: w115 -> [w125 _]
          frame No Error {
            n236 = node-c288() -> (w134:T3)  [unwired: 4 in]
            n237 = timed-loop {
              tunnel: w132 -> [w148]
              tunnel: w127 -> [w147]
              tunnel: [w146] -> w131
              tunnel: [w145] -> w130
              tunnel: [w137] -> w129
              shift-right: [w139] -> _
              shift-left: FALSE -> [w142]
              timing: w134 -> [_]
              timing-out: [_] -> w133
              tunnel: w126 -> [w136]
              tunnel: w125 -> [w135]
              stop <- w143 stop-if-true
              n238 = node-c288() -> ()  [unwired: 1 in, 1 out]
              n239 = Dequeue Element(queue=w136, error in (no error)=w135) -> (element=w138:string)  [unwired: 1 in, 3 out]
              n240 = Select(t=FALSE, s=w142, f=TRUE) -> (s? t:f=w139:bool)
              "TCP packet\nSend To SEPTIC" <- w139
              n241 = TCP Write(connection ID=w148, data in=w138, error in (no error)=w147) -> (connection ID out=w146:refnum<k5>, error out=w145:errorcluster)  [unwired: 1 in, 1 out]
              n242 = local read "stop"() -> (w137:bool)
              n243 = Unbundle(w145) -> ("status"=w144:bool)  [unwired: 2 out]
              n244 = node-c288() -> ()  [unwired: 1 in, 1 out]
              n245 = Compound Arithmetic op=OR(w144, w137) -> (w143:bool)
            }
            n246 = node-c288(w133) -> ()  [unwired: 1 out]
          }
          frame Error {
            n247 = local read "stop"() -> (w153:bool)
          }
        }
        n248 = TCP Close Connection(connection ID=w121, error in (no error)=w120) -> (error out=→"SEPTIC TCP Error Out":errorcluster)  [unwired: 1 in, 1 out]
        n249 = Wait (ms)(milliseconds to wait=u32 1000) -> ()  [unwired: 1 out]
      }
      n250 = node-c288(w46) -> ()  [unwired: 1 out]
    }
    frame Error {
    }
  }
  n251 = VISA Close(VISA resource name=w25, error in (no error)=w26) -> (error out=→"Serial error out":errorcluster)
